vi "取直线亮度与高斯拟合.vi"(6 "拟合方法":T1 items=["Least Square", "Least Absolute Residual", "Bisquare"], 8 "error in":errorcluster, 9 "X":dbl[](array[numeric]), 10 "所在直线":sgl[](array[numeric]), 11 "Image in":T2) -> (0 "error out":errorcluster, 1 "半径um":dbl, 2 "高斯拟合":dbl[](array[numeric]), 3 "原曲线":dbl[](array[numeric]))   [LabVIEW 2015]
uses:
  <vilib>/vision/Image Controls.llb/IMAQ Image.ctl
  <vilib>/Analysis/6fits.llb/Curve Fitting Criteria.ctl
  <vilib>/vision/NI_Vision_Development_Module.lvlib
  <vilib>/Analysis/NI_AALPro.lvlib
panel:
  out "Waveform Graph":dbl[](graph)
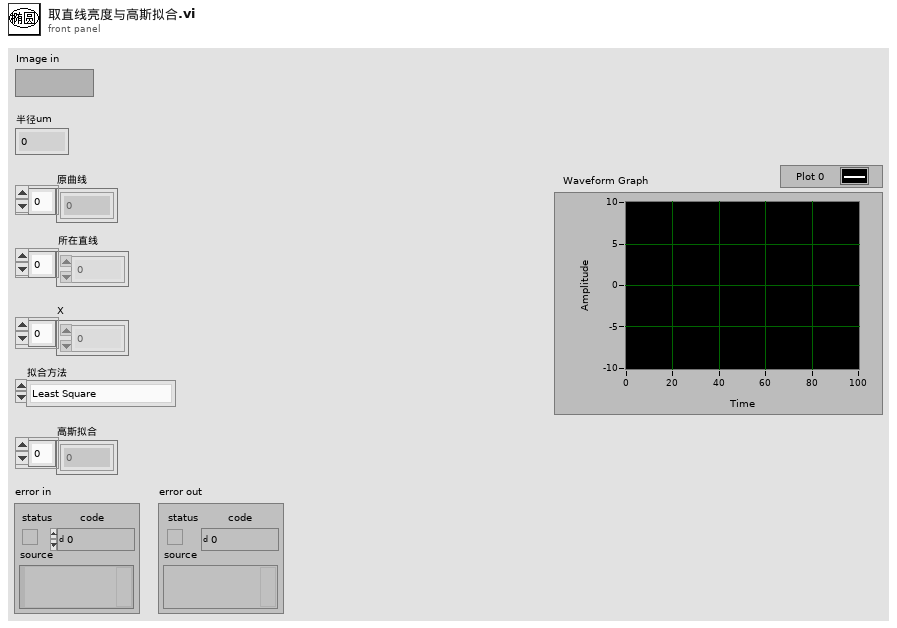
[diagram p1: front panel]
types:
  T1 = typedef "NI_AALPro.lvlib/Curve Fitting Criteria.ctl" = u16
  T2 = typedef "IMAQ Image.ctl" = refnum<image>
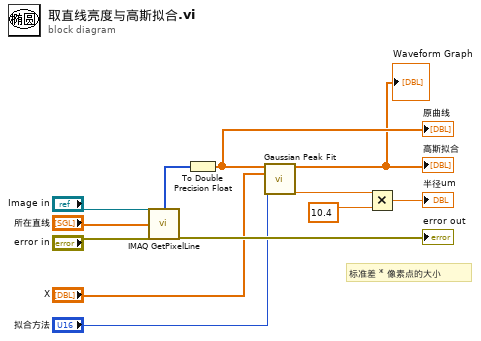
[diagram p0: block diagram]
diagram:
  # "标准差 * 像素点的大小"
  n1 = call "IMAQ GetPixelLine"("error in (no error)"="error in", "Line Coordinates"="所在直线", "Image"="Image in") -> ("error out"=→"error out":errorcluster, "Pixels Line (U8)"=w12:u8[])  [unwired: 1 in, 3 out]
  n2 = To Double Precision Float(number=w12) -> (double precision float=w3:dbl[])
  "原曲线" <- w3
  n3 = call <vilib>:"Gaussian Peak Fit.vi"("Y"=w3, "X"="X", "method"="拟合方法") -> ("Best Gaussian Fit"=→"高斯拟合" →"Waveform Graph":dbl[], "standard deviation"=w6:dbl)  [unwired: 6 in, 5 out]
  n4 = Multiply(x=w6, y=10.4) -> (x*y=→"半径um":dbl)
